vi "art联动采集V4.6.vi"() -> ()   [LabVIEW 2016]
uses:
  <vilib>/Instr/_visa.llb/VISA Configure Serial Port (Instr).vi
  <vilib>/Utility/file.llb/Write Delimited Spreadsheet (DBL).vi
panel:
  in  "分层图查看":bool
  in  "hDevice 2":i32
  in  "逐行扫描":bool
  in  "定位模式":bool
  in  "X终点":dbl
  in  "Y终点":dbl
  in  "高级设置":bool
  in  "Y轴回零速度":dbl=15000.0
  in  "X轴回零速度":dbl=15000.0
  in  "细分设置":dbl=8.0
  in  "等待时间":u32=40
  in  "文件保存":path=path "C:/Users/H301/Desktop/art采集实验数据" caption="保存路径"
  out "行用时（s）":dbl
  out "time（行）":u32
  out "error out":errorcluster caption="错误输出"
  in  "退出扫描(Esc)":bool
  in  "N_Length":i32=16384
  out "M_Length":i32
  out "hDevice":i32=241832032
  out "pulDDR2Length":u32=256
  out "总用时（s）":dbl
  out "毫秒计时值":u32=3586537
  out "数组":dbl[][](array[numeric])=[[58819.77200735986, 88200.32943600747]]
  out "强度图":dbl[][](graph)=[[58819.77200735986, 88200.32943600747]]
  out "judge":dbl
  out "Xloop":dbl
  out "幅频谱":dbl[](graph)
  out "时域谱":dbl[](graph)
  out "错误输出":errorcluster
  in  "启动":bool
  in  "逐点扫描":bool
  in  "X归零":bool
  in  "Y归零":bool
  in  "Y起点":dbl
  in  "Y轴速度":dbl=9000.0
  in  "X轴速度":dbl=9000.0
  out "电机状态":bool
  in  "电机端口":refnum<visa-resource-name>="COM6"
  out "Yloop":dbl=1.0
  out "X扫描范围":dbl=150.0
  out "Y扫描范围":dbl=75.0
  out "Y序":i32
  in  "X起点":dbl
  out "Y(mm)":dbl
  out "x+y 2":dbl=3.0
  in  "Y:":dbl=1.0
  in  "精度":dbl=0.001
  in  "电机急停":bool
  out "X（mm）":dbl
  out "x+y":dbl=1.0
  in  "X:":dbl=1.0
  # "实时坐标"
  # "时域谱"
  # "频域谱"
  # "归零"
  # "扫描区域"
  # "扫描步进(mm)"
  # "X:"
  # "~"
  # "Y:"
  # "~"
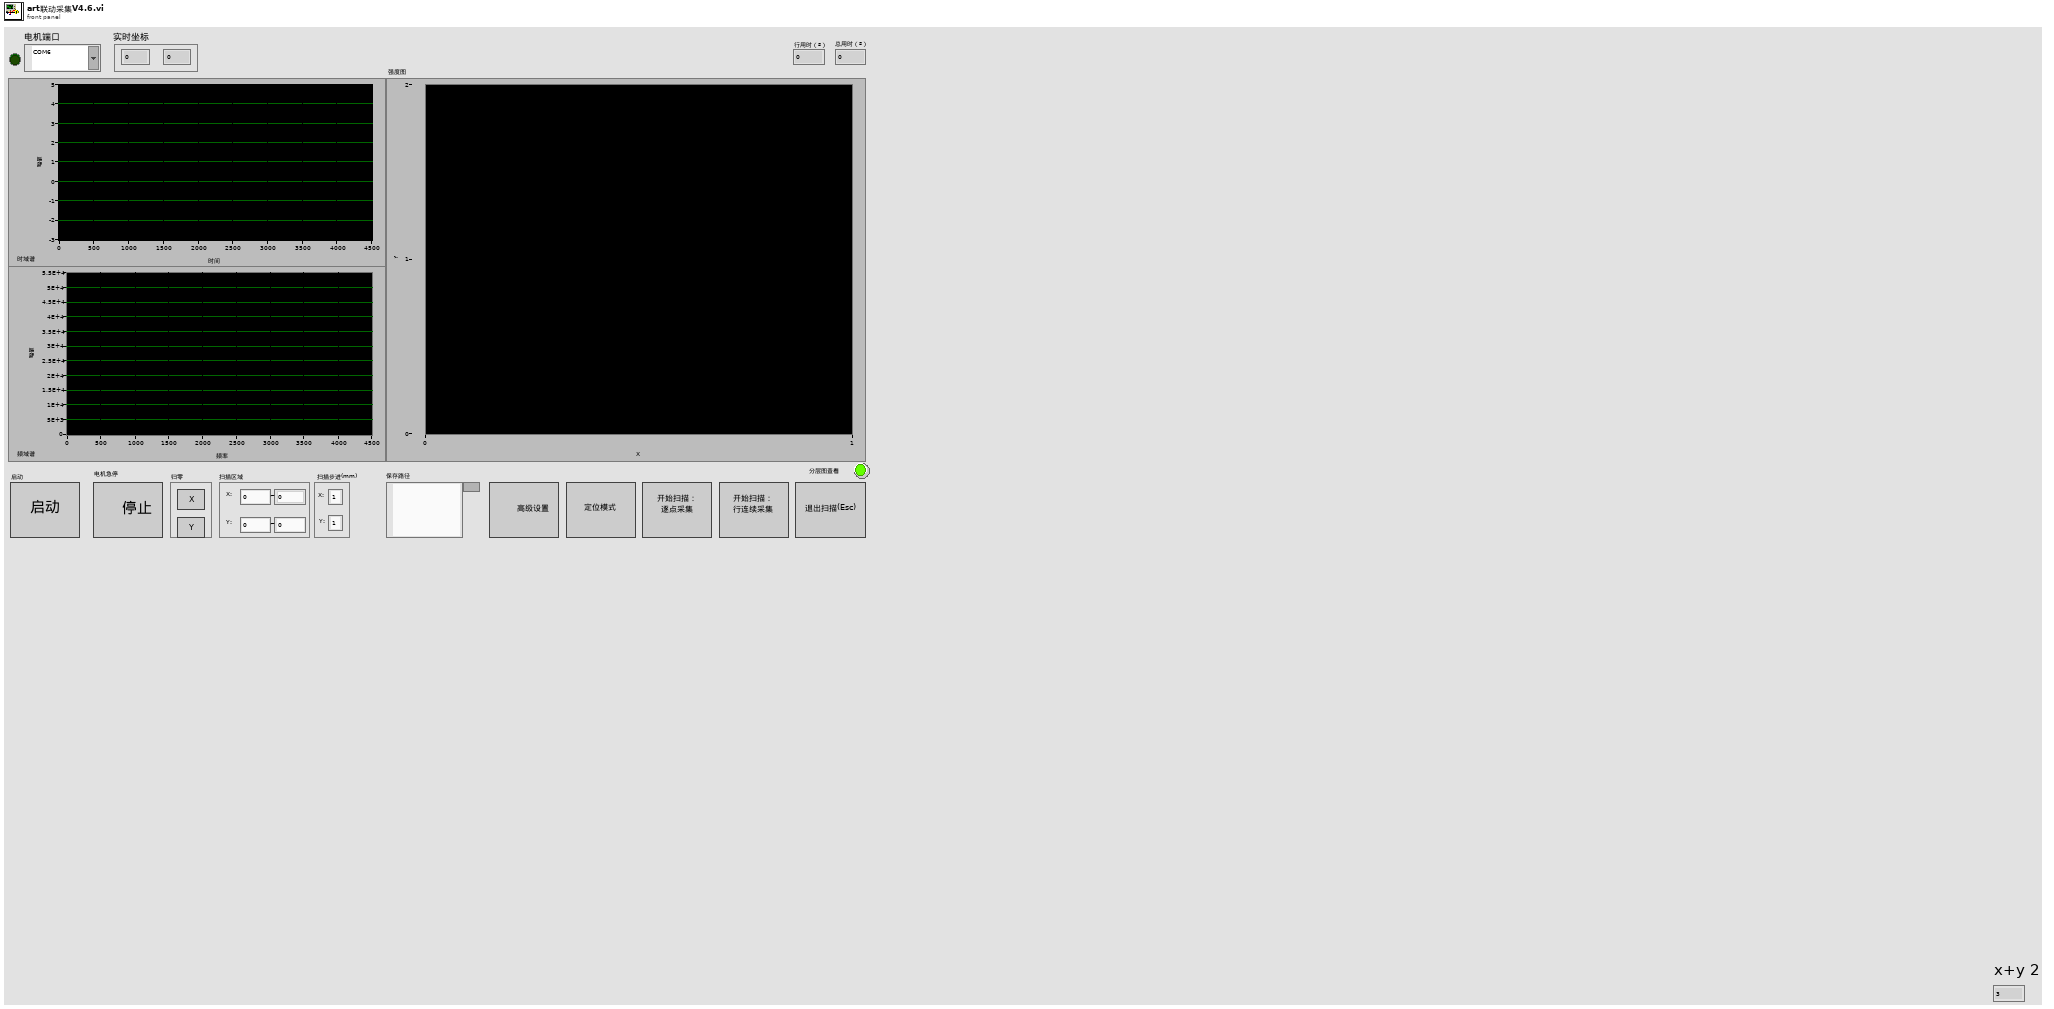
[diagram p1: front panel]
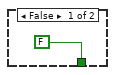
[diagram p2: hidden frame]
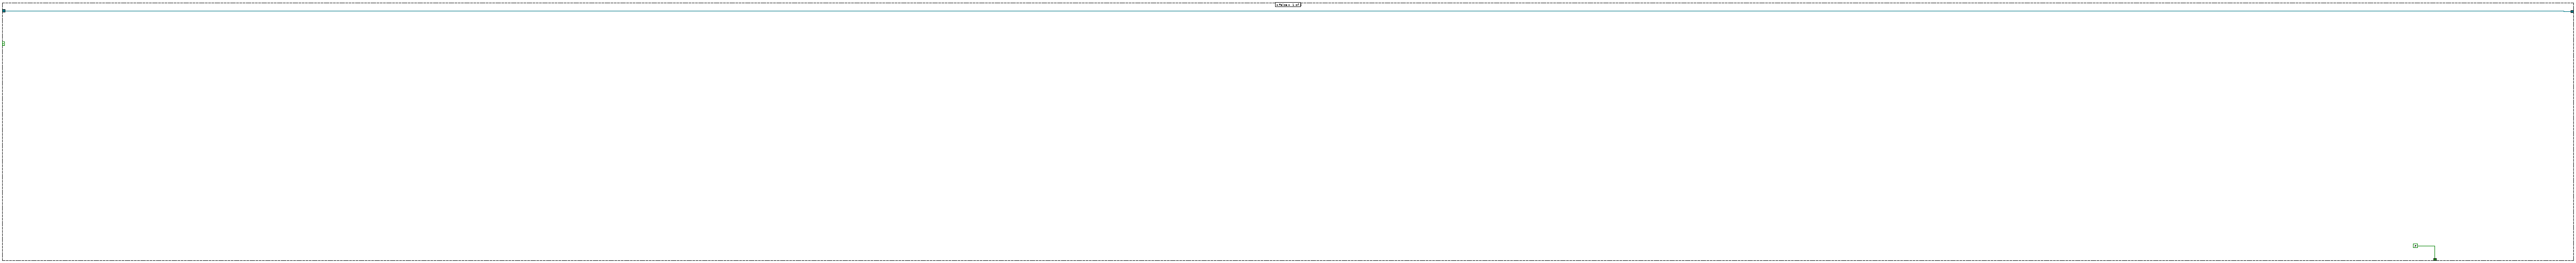
[diagram p3: hidden frame]
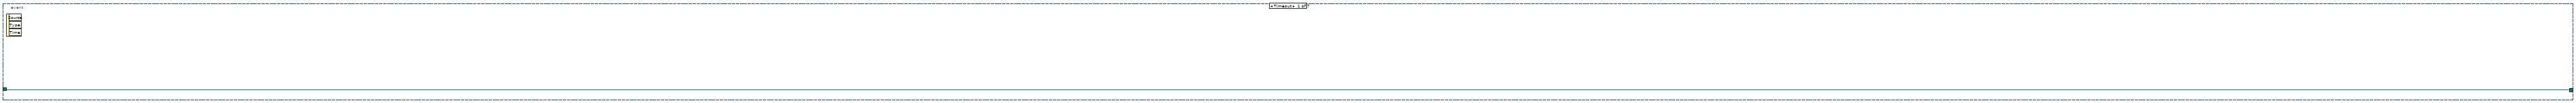
[diagram p4: hidden frame]
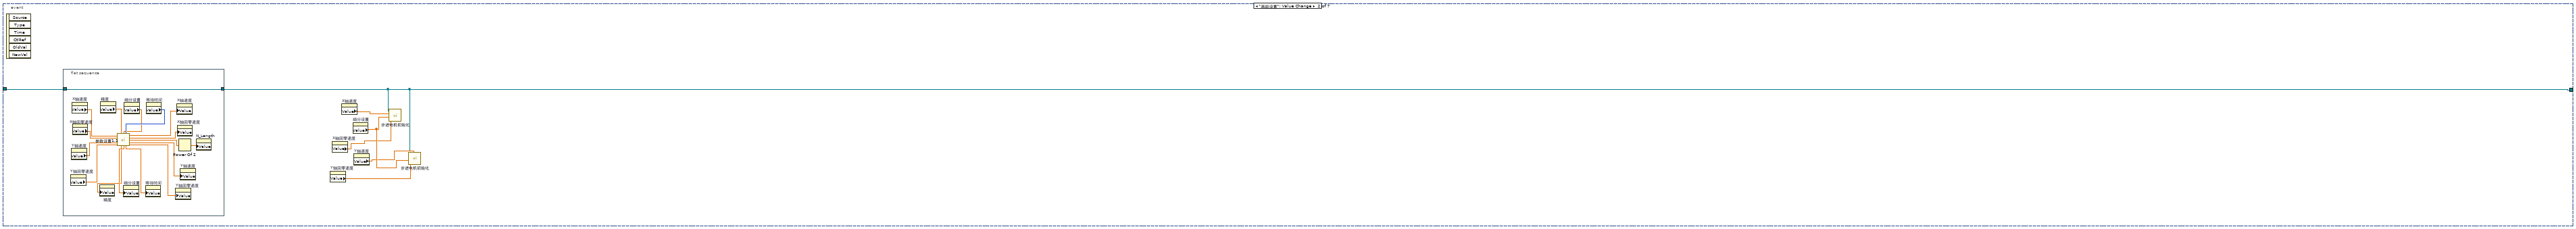
[diagram p5: hidden frame]
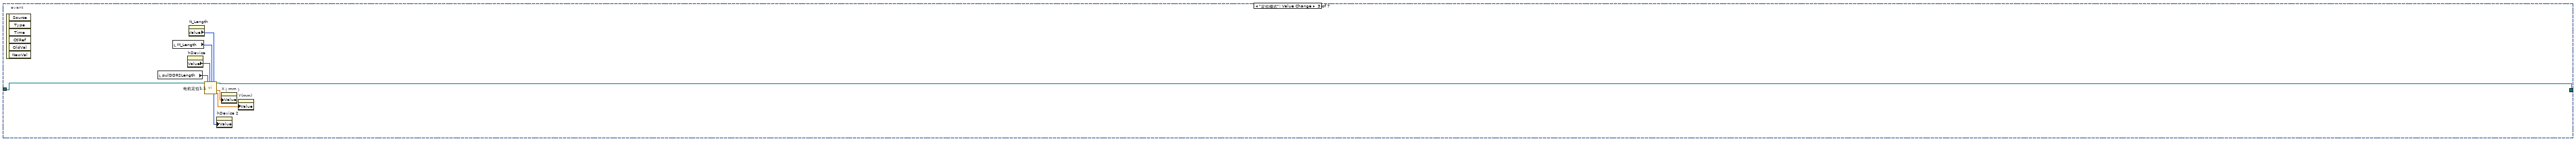
[diagram p6: hidden frame]
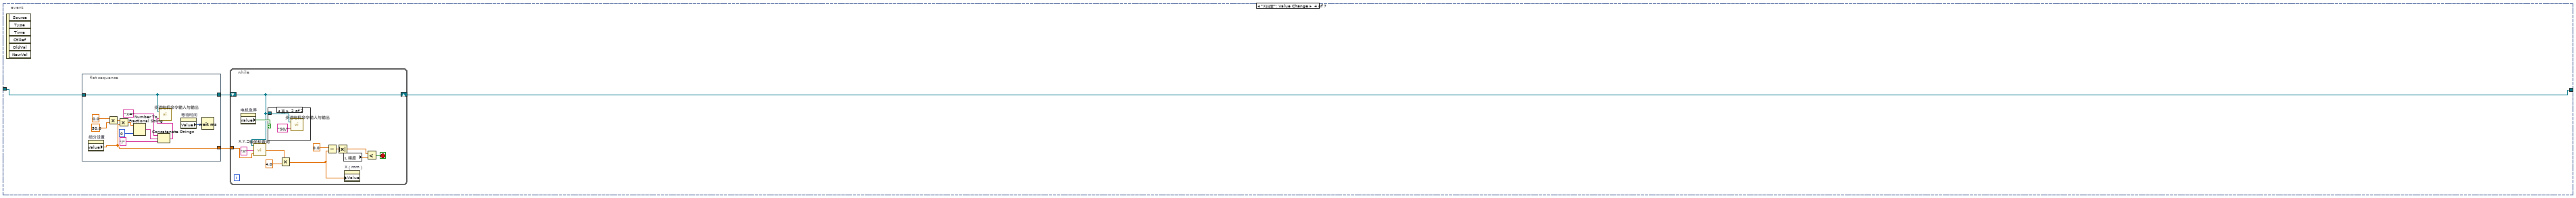
[diagram p7: hidden frame]
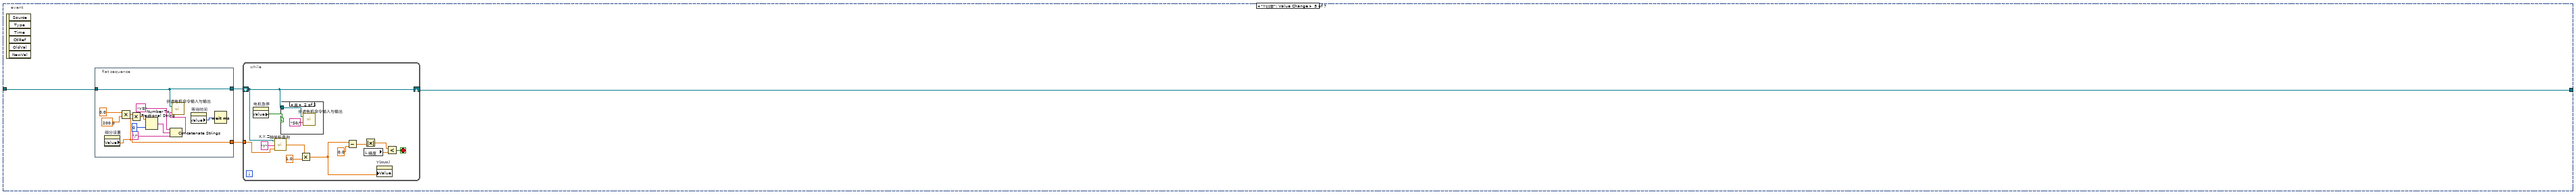
[diagram p9: hidden frame]
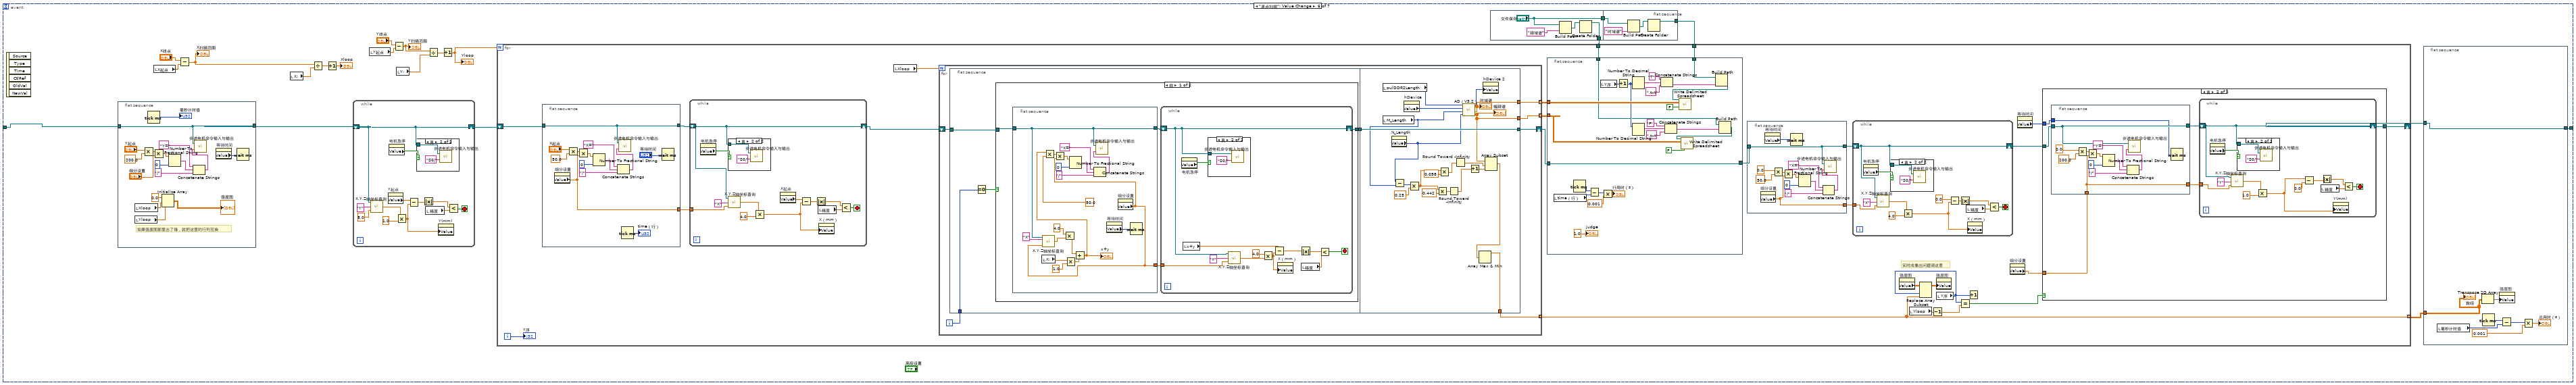
[diagram p11: hidden frame]
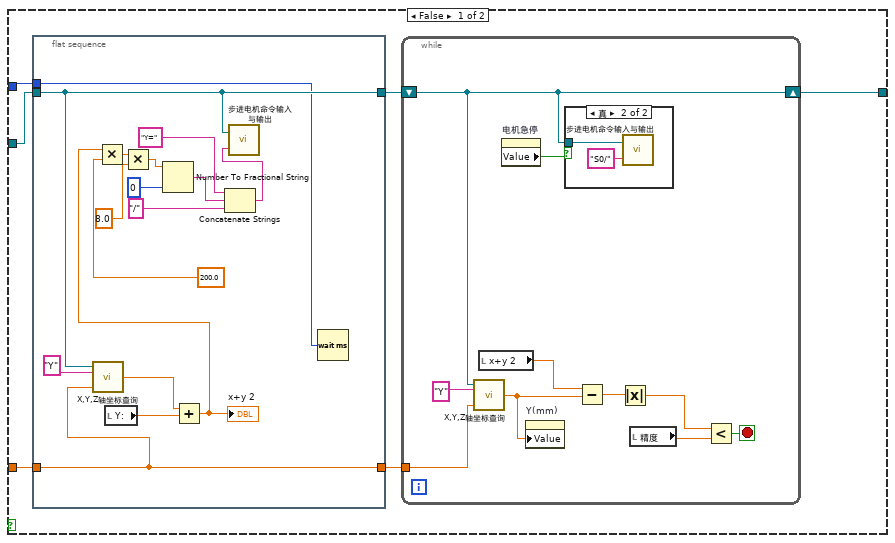
[diagram p15: hidden frame]
diagram:
  n1 = for {
    N: 255 -> [_]
    tunnel: [w10] -> w7 mode=indexing
    i -> [w10]
  }
  n2 = To Unsigned Byte Integer(number=w7) -> (unsigned 8bit integer=w4:u8[])
  n3 = Join Numbers(hi=u16 0, lo=w4) -> ((hi.lo)=w6:u32[])
  n4 = Join Numbers(hi=w4, lo=w4) -> ((hi.lo)=w3:u16[])
  n5 = Join Numbers(hi=w6, lo=w3) -> ((hi.lo)=w2:u64[])
  n6 = property on="强度图" class="IntGraph (严格)"("Color Table"=w2) -> ()  [unwired: 2 in, 2 out]
  n7 = while {
    stop <- w11 stop-if-true
    n8 = case shown="真" "启动" {
      tunnel: [FALSE ("ESC") w20] -> w11
      frame False {
      }
      frame True {
        w33 = 0  # OutClockSource
        w34 = 0  # bClockSourceDir
        w36 = 10000000  # Frequency
        w37 = 0  # ClockSource
        w38 = 0  # TrigLevelVolt
        w26 = 1
        w39 = 0  # TriggerDir
        w40 = 0  # TriggerSource
        w41 = 0  # ATRTriggerChannel
        w42 = 0  # TriggerMode
        w27 = 0  # M_Length
        w43 = 1  # CouplingType
        w44 = 0  # DeviceLgcID
        w54 = u16 0 items=["无", "XON/XOFF", "RTS/CTS", "XON/XOFF & RTS/CTS", "DTR/DSR", "XON/XOFF & DTR/DSR"] ("flow control (0:none)")
        w55 = u16 10 items=["1.0"=10, "1.5"=15, "2.0"=20] ("stop bits (10: 1 bit)")
        # "3"
        # "2"
        # "1"
        n9 = call-poly "VISA Configure Serial Port"("VISA resource name"="电机端口", "baud rate (9600)"=u32 9600, "data bits (8)"=u16 8, "parity (0:none)"=enum16{"None", "Odd", "Even", "Mark", "Space"}."None", "stop bits (10: 1 bit)"=w55, "flow control (0:none)"=w54) -> ("VISA resource name out"=w46:refnum<visa-resource-name>, "error out"=→"error out":errorcluster)  [unwired: 1 in, 7 out]
        n10 = Build Array "InputRange"(w26, w26, w26, w26) -> (w25:i32[])
        n11 = dll-call lib="PTH2aabs CUsersH301Desktopart闭环扫描程序采集卡控制INFamd64PCI8502_32.dll" fn="PCI8502_CreateDevice" label="CreateDevice"("DeviceLgcID"=w44) -> (w31:i32)  [unwired: 4 in, 2 out]
        n12 = property on="细分设置" class="DigNum (严格)"() -> ("Value"=w19:dbl)  [unwired: 2 in, 2 out]
        n13 = Build Array (concatenate) "InitDeviceAD"(w36, w25, w43, w27, "N_Length", w42, w41, w40, w39, w38, w37, w34, w33) -> (w35:i32[])
        n14 = call "步进电机初始化.vi"("回零速度"="X轴回零速度", "细分设置"=w19, "X轴速度"="X轴速度", "串口通信端口"=w46) -> ()  [unwired: 2 in, 1 out]
        n15 = dll-call lib="PTH2aabs CUsersH301Desktopart闭环扫描程序采集卡控制INFamd64PCI8502_32.dll" fn="PCI8502_GetDDR2Length" label="GetDDR2Length"("hDevice"=w31, "pulDDR2Length"=u32 0) -> ("hDevice"=w30:i32, "pulDDR2Length"=→"pulDDR2Length":u32)  [unwired: 4 in, 2 out]
        n16 = call "步进电机初始化.vi"("Y轴速度"="Y轴速度", "回零速度"="Y轴回零速度", "细分设置"=w19, "串口通信端口"=w46) -> ()  [unwired: 2 in, 1 out]
        n17 = call "步进电机命令输入与输出.vi"("输入字符串"="?R/", "串口通信端口"=w46) -> ("返回字符串"=w51:string)
        n18 = dll-call lib="PTH2aabs CUsersH301Desktopart闭环扫描程序采集卡控制INFamd64PCI8502_32.dll" fn="PCI8502_InitDeviceAD" label="InitDeviceAD"("hDevice"=w30, "pADPara"=w35) -> ("hDevice"=→"hDevice":i32)  [unwired: 5 in, 2 out]
        n19 = String Subset(string=w51, offset (0)=0 ("偏移量(0)"), length (rest)=2 ("长度（剩余）")) -> (substring=w48:string)
        n20 = Equal?(x=w48, y="OK") -> (x = y?=w45:bool)
        "电机状态" <- w45
        n21 = case shown="真" w45 {
          tunnel: w46 -> [w61 w64]
          tunnel: [w61 w62] -> w21
          tunnel: [FALSE ("ESC") w63] -> w20
          frame False {
          }
          frame True {
            n22 = while {
              tunnel: ["退出扫描(Esc)"] -> w63
              shift-right: [w65] -> w62
              shift-left: w64 -> [w70]
              stop <- "退出扫描(Esc)" stop-if-true
              n23 = property on="高级设置" class="Bool"("Visible"=TRUE ("可见")) -> ()  [unwired: 2 in, 2 out]
              n24 = property on="定位模式" class="Bool"("Visible"=TRUE ("可见")) -> ()  [unwired: 2 in, 2 out]
              n25 = event shown="[6] \"分层图查看\": 值改变" {
                selector: _ -> [_ _ _ _ _ _ _]
                dyn-events: _ -> [_ _ _ _ _ _ _]
                timeout: 1 -> [_ _ _ _ _ _ _]
                tunnel: w70 -> [w71 w78 w104 w108 w138 w185 w472]
                tunnel: [w71 w72 w103 w106 w136 w179 w471] -> w65
                event Timeout {
                  n26 = event-data() -> ()  [unwired: 1 in, 3 out]
                }
                event "高级设置": Value Change {
                  n27 = event-data() -> ()  [unwired: 1 in, 6 out]
                  n28 = flat-sequence {
                    tunnel: w78 -> [w81]
                    tunnel: [w81] -> w72
                    frame #0 {
                      n29 = property on="Y轴回零速度" class="DigNum (严格)"() -> ("Value"=w85:dbl)  [unwired: 2 in, 2 out]
                      n30 = property on="Y轴速度" class="DigNum (严格)"() -> ("Value"=w84:dbl)  [unwired: 2 in, 2 out]
                      n31 = property on="X轴速度" class="DigNum (严格)"() -> ("Value"=w82:dbl)  [unwired: 2 in, 2 out]
                      n32 = property on="X轴回零速度" class="DigNum (严格)"() -> ("Value"=w83:dbl)  [unwired: 2 in, 2 out]
                      n33 = property on="精度" class="DigNum (严格)"() -> ("Value"=w89:dbl)  [unwired: 2 in, 2 out]
                      n34 = property on="细分设置" class="DigNum (严格)"() -> ("Value"=w90:dbl)  [unwired: 2 in, 2 out]
                      n35 = property on="等待时间" class="DigNum (严格)"() -> ("Value"=w91:u32)  [unwired: 2 in, 2 out]
                      n36 = call "参数设置1.1.vi"("X轴速度"=w82, "精度"=w89, "细分设置"=w90, "等待时间"=w91, "X轴回零速度"=w83, "Y轴速度"=w84, "Y轴回零速度"=w85) -> ("X轴速度"=w92:dbl, "X轴回零速度"=w93:dbl, "采样阶"=w79:dbl, "Y轴速度"=w94:dbl, "精度"=w86:dbl, "细分设置"=w87:dbl, "等待时间"=w88:dbl, "Y轴回零速度"=w95:dbl)  [unwired: 1 in]
                      n37 = property on="精度" class="DigNum (严格)"("Value"=w86) -> ()  [unwired: 2 in, 2 out]
                      n38 = property on="细分设置" class="DigNum (严格)"("Value"=w87) -> ()  [unwired: 2 in, 2 out]
                      n39 = property on="等待时间" class="DigNum (严格)"("Value"=w88) -> ()  [unwired: 2 in, 2 out]
                      n40 = property on="Y轴回零速度" class="DigNum (严格)"("Value"=w95) -> ()  [unwired: 2 in, 2 out]
                      n41 = property on="X轴速度" class="DigNum (严格)"("Value"=w92) -> ()  [unwired: 2 in, 2 out]
                      n42 = property on="X轴回零速度" class="DigNum (严格)"("Value"=w93) -> ()  [unwired: 2 in, 2 out]
                      n43 = Power Of 2(x=w79) -> (2^x=w80:dbl)
                      n44 = property on="Y轴速度" class="DigNum (严格)"("Value"=w94) -> ()  [unwired: 2 in, 2 out]
                      n45 = property on="N_Length" class="DigNum (严格)"("Value"=w80) -> ()  [unwired: 2 in, 2 out]
                    }
                  }
                  n46 = property on="Y轴回零速度" class="DigNum (严格)"() -> ("Value"=w74:dbl)  [unwired: 2 in, 2 out]
                  n47 = property on="X轴回零速度" class="DigNum (严格)"() -> ("Value"=w75:dbl)  [unwired: 2 in, 2 out]
                  n48 = property on="X轴速度" class="DigNum (严格)"() -> ("Value"=w76:dbl)  [unwired: 2 in, 2 out]
                  n49 = property on="细分设置" class="DigNum (严格)"() -> ("Value"=w77:dbl)  [unwired: 2 in, 2 out]
                  n50 = property on="Y轴速度" class="DigNum (严格)"() -> ("Value"=w73:dbl)  [unwired: 2 in, 2 out]
                  n51 = call "步进电机初始化.vi"("回零速度"=w75, "细分设置"=w77, "X轴速度"=w76, "串口通信端口"=w72) -> ()  [unwired: 2 in, 1 out]
                  n52 = call "步进电机初始化.vi"("Y轴速度"=w73, "回零速度"=w74, "细分设置"=w77, "串口通信端口"=w72) -> ()  [unwired: 2 in, 1 out]
                }
                event "定位模式": Value Change {
                  n53 = event-data() -> ()  [unwired: 1 in, 6 out]
                  n54 = local read "pulDDR2Length"() -> (w100:u32)
                  n55 = local read "M_Length"() -> (w98:i32)
                  n56 = property on="hDevice" class="DigNum (严格)"() -> ("Value"=w99:i32)  [unwired: 2 in, 2 out]
                  n57 = property on="N_Length" class="DigNum (严格)"() -> ("Value"=w97:i32)  [unwired: 2 in, 2 out]
                  n58 = call "电机定位1.1.vi"("VISA I"=w104, "pulDDR2Length"=w100, "hDevice"=w99, "M-length"=w98, "N-length"=w97) -> ("hDevice out"=w96:i32, "VISA O"=w103:refnum<visa-resource-name>, "X"=w102:dbl, "Y"=w101:dbl)  [unwired: 11 in]
                  n59 = property on="hDevice 2" class="DigNum (严格)"("Value"=w96) -> ()  [unwired: 2 in, 2 out]
                  n60 = property on="X（mm）" class="DigNum (严格)"("Value"=w102) -> ()  [unwired: 2 in, 2 out]
                  n61 = property on="Y(mm)" class="DigNum (严格)"("Value"=w101) -> ()  [unwired: 2 in, 2 out]
                }
                event "X归零": Value Change {
                  n62 = event-data() -> ()  [unwired: 1 in, 6 out]
                  n63 = flat-sequence {
                    tunnel: w108 -> [w112]
                    tunnel: [w112] -> w107
                    tunnel: [w109] -> w105
                    frame #0 {
                      n64 = property on="细分设置" class="DigNum (严格)"() -> ("Value"=w109:dbl)  [unwired: 2 in, 2 out]
                      n65 = Multiply(x=0.0, y=50.0) -> (x*y=w115:dbl)
                      n66 = Multiply(x=w115, y=w109) -> (x*y=w120:dbl)
                      n67 = Number To Fractional String(number=w120, precision (6)=i16 0 ("精度(6)")) -> (F-format string=w118:string)  [unwired: 2 out]
                      n68 = Concatenate Strings("X=" ("字符串"), w118, "/" ("字符串")) -> (w113:string)
                      n69 = call "步进电机命令输入与输出.vi"("输入字符串"=w113, "串口通信端口"=w112) -> ()  [unwired: 1 out]
                      n70 = property on="等待时间" class="DigNum (严格)"() -> ("Value"=w110:u32)  [unwired: 2 in, 2 out]
                      n71 = Wait (ms)(milliseconds to wait=w110) -> ()  [unwired: 1 out]
                    }
                  }
                  n72 = while {
                    tunnel: w105 -> [w121]
                    shift-right: [w122] -> w106
                    shift-left: w107 -> [w122]
                    stop <- w128 stop-if-true
                    n73 = property on="电机急停" class="Bool (严格)"() -> ("Value"=w129:bool)  [unwired: 2 in, 2 out]
                    n74 = call "X,Y,Z轴坐标查询.vi"("细分设置"=w121, "查询坐标轴"="X", "串口通信端口"=w122) -> ("坐标(mm)"=w130:dbl)
                    n75 = case shown="真" w129 {
                      tunnel: w122 -> [_ w133]
                      frame False {
                      }
                      frame True {
                        n76 = call "步进电机命令输入与输出.vi"("输入字符串"="S0/", "串口通信端口"=w133) -> ()  [unwired: 1 out]
                      }
                    }
                    n77 = Multiply(x=w130, y=4.0 ("x")) -> (x*y=w126:dbl)
                    n78 = Subtract(x=0.0, y=w126) -> (x-y=w125:dbl)
                    n79 = Absolute Value(x=w125) -> (abs(x)=w124:dbl)
                    n80 = local read "精度"() -> (w127:dbl)
                    n81 = property on="X（mm）" class="DigNum (严格)"("Value"=w126) -> ()  [unwired: 2 in, 2 out]
                    n82 = Less?(x=w124, y=w127) -> (x < y?=w128:bool)
                  }
                }
                event "Y归零": Value Change {
                  n83 = event-data() -> ()  [unwired: 1 in, 6 out]
                  n84 = flat-sequence {
                    tunnel: w138 -> [w142]
                    tunnel: [w142] -> w137
                    tunnel: [w139] -> w135
                    frame #0 {
                      n85 = property on="细分设置" class="DigNum (严格)"() -> ("Value"=w139:dbl)  [unwired: 2 in, 2 out]
                      n86 = Multiply(x=0.0, y=200.0) -> (x*y=w145:dbl)
                      n87 = Multiply(x=w145, y=w139) -> (x*y=w150:dbl)
                      n88 = Number To Fractional String(number=w150, precision (6)=i16 0 ("精度(6)")) -> (F-format string=w148:string)  [unwired: 2 out]
                      n89 = Concatenate Strings("Y=" ("字符串"), w148, "/" ("字符串")) -> (w143:string)
                      n90 = call "步进电机命令输入与输出.vi"("输入字符串"=w143, "串口通信端口"=w142) -> ()  [unwired: 1 out]
                      n91 = property on="等待时间" class="DigNum (严格)"() -> ("Value"=w140:u32)  [unwired: 2 in, 2 out]
                      n92 = Wait (ms)(milliseconds to wait=w140) -> ()  [unwired: 1 out]
                    }
                  }
                  n93 = while {
                    tunnel: w135 -> [w151]
                    shift-right: [w152] -> w136
                    shift-left: w137 -> [w152]
                    stop <- w158 stop-if-true
                    n94 = property on="电机急停" class="Bool (严格)"() -> ("Value"=w159:bool)  [unwired: 2 in, 2 out]
                    n95 = call "X,Y,Z轴坐标查询.vi"("细分设置"=w151, "查询坐标轴"="Y", "串口通信端口"=w152) -> ("坐标(mm)"=w160:dbl)
                    n96 = case shown="真" w159 {
                      tunnel: w152 -> [_ w163]
                      frame False {
                      }
                      frame True {
                        n97 = call "步进电机命令输入与输出.vi"("输入字符串"="S0/", "串口通信端口"=w163) -> ()  [unwired: 1 out]
                      }
                    }
                    n98 = Multiply(x=w160, y=1.0 ("x")) -> (x*y=w156:dbl)
                    n99 = Subtract(x=w156, y=0.0 ("x")) -> (x-y=w154:dbl)
                    n100 = local read "精度"() -> (w157:dbl)
                    n101 = Absolute Value(x=w154) -> (abs(x)=w153:dbl)
                    n102 = property on="Y(mm)" class="DigNum (严格)"("Value"=w156) -> ()  [unwired: 2 in, 2 out]
                    n103 = Less?(x=w153, y=w157) -> (x < y?=w158:bool)
                  }
                }
                event "逐点扫描": Value Change {
                  n104 = event-data() -> ()  [unwired: 1 in, 6 out]
                  n105 = flat-sequence {
                    tunnel: w185 -> [w210]
                    tunnel: [w210] -> w175
                    frame #0 {
                      # "如果强度图那里出了错，就把这里的行列互换"
                      n106 = local read "Xloop"() -> (w205:dbl)
                      n107 = local read "Yloop"() -> (w204:dbl)
                      n108 = Multiply(x="Y起点", y=200.0) -> (x*y=w213:dbl)
                      n109 = Tick Count (ms)() -> (millisecond timer value=→"毫秒计时值":u32)
                      n110 = Multiply(x=w213, y="细分设置") -> (x*y=w218:dbl)
                      n111 = Initialize Array(0.0 ("元素"), w205, w204) -> (→"强度图":dbl[][])
                      n112 = Number To Fractional String(number=w218, precision (6)=i16 0 ("精度(6)")) -> (F-format string=w216:string)  [unwired: 2 out]
                      n113 = Concatenate Strings("Y=" ("字符串"), w216, "/" ("字符串")) -> (w211:string)
                      n114 = call "步进电机命令输入与输出.vi"("输入字符串"=w211, "串口通信端口"=w210) -> ()  [unwired: 1 out]
                      n115 = property on="等待时间" class="DigNum (严格)"() -> ("Value"=w202:u32)  [unwired: 2 in, 2 out]
                      n116 = Wait (ms)(milliseconds to wait=w202) -> ()  [unwired: 1 out]
                    }
                  }
                  n117 = local read "X起点"() -> (w171:dbl)
                  n118 = Subtract(x="X终点", y=w171) -> (x-y=w170:dbl)
                  "X扫描范围" <- w170
                  n119 = local read "X:"() -> (w178:dbl)
                  n120 = Divide(x=w170, y=w178) -> (x/y=w176:dbl)
                  n121 = Increment(x=w176) -> (x+1=→"Xloop":dbl)
                  n122 = while {
                    shift-right: [w219] -> w167
                    shift-left: w175 -> [w219]
                    stop <- w224 stop-if-true
                    n123 = call "X,Y,Z轴坐标查询.vi"("细分设置"=8.0, "查询坐标轴"="Y", "串口通信端口"=w219) -> ("坐标(mm)"=w226:dbl)
                    n124 = property on="Y起点" class="DigNum (严格)"() -> ("Value"=w228:dbl)  [unwired: 2 in, 2 out]
                    n125 = property on="电机急停" class="Bool (严格)"() -> ("Value"=w225:bool)  [unwired: 2 in, 2 out]
                    n126 = Multiply(x=w226, y=1.0 ("x")) -> (x*y=w222:dbl)
                    n127 = Subtract(x=w228, y=w222) -> (x-y=w221:dbl)
                    n128 = case shown="真" w225 {
                      tunnel: w219 -> [_ w231]
                      frame False {
                      }
                      frame True {
                        n129 = call "步进电机命令输入与输出.vi"("输入字符串"="S0/", "串口通信端口"=w231) -> ()  [unwired: 1 out]
                      }
                    }
                    n130 = Absolute Value(x=w221) -> (abs(x)=w220:dbl)
                    n131 = local read "精度"() -> (w223:dbl)
                    n132 = property on="Y(mm)" class="DigNum (严格)"("Value"=w222) -> ()  [unwired: 2 in, 2 out]
                    n133 = Less?(x=w220, y=w223) -> (x < y?=w224:bool)
                  }
                  n134 = local read "Y起点"() -> (w173:dbl)
                  n135 = Subtract(x="Y终点", y=w173) -> (x-y=w169:dbl)
                  "Y扫描范围" <- w169
                  n136 = local read "Y:"() -> (w184:dbl)
                  n137 = Divide(x=w169, y=w184) -> (x/y=w183:dbl)
                  n138 = Increment(x=w183) -> (x+1=w182:dbl)
                  "Yloop" <- w182
                  n139 = for {
                    N: w182 -> [_]
                    shift-right: [w255] -> w181
                    shift-left: w167 -> [w235]
                    tunnel: [w237] -> w180 mode=indexing
                    tunnel: w165 -> [w241]
                    tunnel: w168 -> [w240]
                    i -> [w256]
                    # "实时成像出问题调这里"
                    n140 = flat-sequence {
                      tunnel: w235 -> [w313]
                      tunnel: [w313] -> w254
                      tunnel: [w309] -> w245
                      frame #0 {
                        n141 = property on="细分设置" class="DigNum (严格)"() -> ("Value"=w309:dbl)  [unwired: 2 in, 2 out]
                        n142 = Multiply(x="X起点", y=50.0) -> (x*y=w316:dbl)
                        n143 = Multiply(x=w316, y=w309) -> (x*y=w321:dbl)
                        n144 = Number To Fractional String(number=w321, precision (6)=i16 0 ("精度(6)")) -> (F-format string=w319:string)  [unwired: 2 out]
                        n145 = Concatenate Strings("X=" ("字符串"), w319, "/" ("字符串")) -> (w314:string)
                        n146 = call "步进电机命令输入与输出.vi"("输入字符串"=w314, "串口通信端口"=w313) -> ()  [unwired: 1 out]
                        n147 = Tick Count (ms)() -> (millisecond timer value=→"time（行）":u32)
                        n148 = Wait (ms)(milliseconds to wait="等待时间") -> ()  [unwired: 1 out]
                      }
                    }
                    n149 = while {
                      tunnel: w245 -> [w323]
                      shift-right: [w322] -> w233
                      shift-left: w254 -> [w322]
                      stop <- w328 stop-if-true
                      n150 = property on="电机急停" class="Bool (严格)"() -> ("Value"=w329:bool)  [unwired: 2 in, 2 out]
                      n151 = case shown="真" w329 {
                        tunnel: w322 -> [_ w334]
                        frame False {
                        }
                        frame True {
                          n152 = call "步进电机命令输入与输出.vi"("输入字符串"="S0/", "串口通信端口"=w334) -> ()  [unwired: 1 out]
                        }
                      }
                      n153 = call "X,Y,Z轴坐标查询.vi"("细分设置"=w323, "查询坐标轴"="X", "串口通信端口"=w322) -> ("坐标(mm)"=w330:dbl)
                      n154 = Multiply(x=w330, y=4.0 ("x")) -> (x*y=w326:dbl)
                      n155 = property on="X起点" class="DigNum (严格)"() -> ("Value"=w332:dbl)  [unwired: 2 in, 2 out]
                      n156 = Subtract(x=w332, y=w326) -> (x-y=w325:dbl)
                      n157 = Absolute Value(x=w325) -> (abs(x)=w324:dbl)
                      n158 = local read "精度"() -> (w327:dbl)
                      n159 = property on="X（mm）" class="DigNum (严格)"("Value"=w326) -> ()  [unwired: 2 in, 2 out]
                      n160 = Less?(x=w324, y=w327) -> (x < y?=w328:bool)
                    }
                    n161 = local read "Xloop"() -> (w246:dbl)
                    n162 = for {
                      N: w246 -> [_]
                      shift-right: [w407] -> w234
                      shift-left: w233 -> [w402]
                      tunnel: [w406] -> w253 mode=indexing
                      tunnel: [w405] -> w252 mode=indexing
                      tunnel: [w404] -> w237 mode=indexing
                      i -> [w403]
                      n163 = flat-sequence {
                        tunnel: w402 -> [w412]
                        tunnel: [w411] -> w408
                        tunnel: w403 -> [w409]
                        tunnel: [w470] -> w407
                        tunnel: w408 -> [w470]
                        tunnel: [w469] -> w406
                        tunnel: [w468] -> w405
                        tunnel: [w466] -> w404
                        frame #0 {
                          n164 = Equal To 0?(x=w409) -> (x = 0?=w410:bool)
                          n165 = case shown="假" w410 {
                            tunnel: w412 -> [w415 w450]
                            tunnel: [w414 w450] -> w411
                            frame False {
                              n166 = flat-sequence {
                                tunnel: w415 -> [w425]
                                tunnel: [w425] -> w416
                                tunnel: [w417] -> w413
                                frame #0 {
                                n167 = local read "X:"() -> (w419:dbl)
                                n168 = Multiply(x=w419, y=1.0 ("x")) -> (x*y=w424:dbl)
                                n169 = property on="等待时间" class="DigNum (严格)"() -> ("Value"=w418:u32)  [unwired: 2 in, 2 out]
                                n170 = property on="细分设置" class="DigNum (严格)"() -> ("Value"=w417:dbl)  [unwired: 2 in, 2 out]
                                n171 = call "X,Y,Z轴坐标查询.vi"("细分设置"=w417, "查询坐标轴"="X", "串口通信端口"=w425) -> ("坐标(mm)"=w421:dbl)
                                n172 = Multiply(x=4.0, y=w421) -> (x*y=w420:dbl)
                                n173 = Add(x=w420, y=w424) -> (x+y=w427:dbl)
                                "x+y" <- w427
                                n174 = Multiply(x=w427, y=50.0) -> (x*y=w430:dbl)
                                n175 = Multiply(x=w430, y=w417) -> (x*y=w435:dbl)
                                n176 = Number To Fractional String(number=w435, precision (6)=i16 0 ("精度(6)")) -> (F-format string=w433:string)  [unwired: 2 out]
                                n177 = Concatenate Strings("X=" ("字符串"), w433, "/" ("字符串")) -> (w428:string)
                                n178 = call "步进电机命令输入与输出.vi"("输入字符串"=w428, "串口通信端口"=w425) -> ()  [unwired: 1 out]
                                n179 = Wait (ms)(milliseconds to wait=w418) -> ()  [unwired: 1 out]
                                }
                              }
                              n180 = while {
                                tunnel: w413 -> [w436]
                                shift-right: [w445] -> w414
                                shift-left: w416 -> [w445]
                                stop <- w444 stop-if-true
                                n181 = property on="电机急停" class="Bool (严格)"() -> ("Value"=w442:bool)  [unwired: 2 in, 2 out]
                                n182 = local read "x+y"() -> (w446:dbl)
                                n183 = case shown="真" w442 {
                                tunnel: w445 -> [_ w448]
                                frame False {
                                }
                                frame True {
                                n184 = call "步进电机命令输入与输出.vi"("输入字符串"="S0/", "串口通信端口"=w448) -> ()  [unwired: 1 out]
                                }
                                }
                                n185 = call "X,Y,Z轴坐标查询.vi"("细分设置"=w436, "查询坐标轴"="X", "串口通信端口"=w445) -> ("坐标(mm)"=w440:dbl)
                                n186 = Multiply(x=4.0, y=w440) -> (x*y=w439:dbl)
                                n187 = Subtract(x=w446, y=w439) -> (x-y=w438:dbl)
                                n188 = property on="X（mm）" class="DigNum (严格)"("Value"=w439) -> ()  [unwired: 2 in, 2 out]
                                n189 = Absolute Value(x=w438) -> (abs(x)=w437:dbl)
                                n190 = local read "精度"() -> (w441:dbl)
                                n191 = Less?(x=w437, y=w441) -> (x < y?=w444:bool)
                              }
                            }
                            frame True {
                            }
                          }
                        }
                        frame #1 {
                          n192 = local read "pulDDR2Length"() -> (w465:u32)
                          n193 = local read "M_Length"() -> (w464:i32)
                          n194 = property on="N_Length" class="DigNum (严格)"() -> ("Value"=w453:i32)  [unwired: 2 in, 2 out]
                          n195 = Subtract(x=w453, y=w464) -> (x-y=w462:i32)
                          n196 = property on="hDevice" class="DigNum (严格)"() -> ("Value"=w451:i32)  [unwired: 2 in, 2 out]
                          n197 = Multiply(x=w462, y=0.25) -> (x*y=w455:dbl)
                          n198 = Multiply(x=w455, y=0.442) -> (x*y=w457:dbl)
                          n199 = Multiply(x=w455, y=0.058) -> (x*y=w459:dbl)
                          n200 = Round Toward -Infinity(1:w457) -> (0:w454:dbl)
                          n201 = Round Toward -Infinity(1:w459) -> (0:w458:dbl)
                          n202 = call "AD（V3.2）.vi"("N-length"=w453, "M-length"=w464, "hDevice"=w451, "pulDDR2Length"=w465) -> ("幅频谱"=w468:dbl[], "时域谱"=w469:dbl[], "hDevice out"=w452:i32)  [unwired: 5 in]
                          "时域谱" <- w469
                          "幅频谱" <- w468
                          n203 = Increment(x=w454) -> (x+1=w461:dbl)
                          n204 = property on="hDevice 2" class="DigNum (严格)"("Value"=w452) -> ()  [unwired: 2 in, 2 out]
                          n205 = Array Subset(array=w468, index=w458, length=w461) -> (w467:dbl[])
                          n206 = Array Max & Min(array=w467) -> (max value=w466:dbl)  [unwired: 3 out]
                        }
                      }
                    }
                    n207 = flat-sequence {
                      tunnel: w252 -> [w290]
                      tunnel: w253 -> [w298]
                      tunnel: w234 -> [w307]
                      tunnel: [w307] -> w248
                      tunnel: w241 -> [w285]
                      tunnel: w240 -> [w284]
                      frame #0 {
                        n208 = local read "time（行）"() -> (w306:u32)
                        n209 = Tick Count (ms)() -> (millisecond timer value=w302:u32)
                        n210 = Subtract(x=w302, y=w306) -> (x-y=w305:u32)
                        n211 = local read "Y序"() -> (w286:i32)
                        n212 = Multiply(x=w305, y=0.001) -> (x*y=→"行用时（s）":dbl)
                        n213 = Increment(x=w286) -> (x+1=w287:i32)
                        n214 = Number To Decimal String(number=w287) -> (decimal integer string=w296:string)  [unwired: 1 in]
                        n215 = Number To Decimal String(number=w287) -> (decimal integer string=w295:string)  [unwired: 1 in]
                        n216 = Concatenate Strings("T" ("字符串"), w296, ".txt" ("字符串")) -> (w299:string)
                        n217 = Concatenate Strings("F" ("字符串"), w295, ".txt" ("字符串")) -> (w293:string)
                        n218 = Build Path(base path=w285, name or relative path=w299) -> (appended path=w301:path)
                        n219 = call-poly <vilib>:"Write Delimited Spreadsheet.vi"("file path (dialog if empty)"=w301, "2D data"=w298, "transpose? (no:F)"=FALSE) -> ()  [unwired: 11 in, 2 out]
                        n220 = Build Path(base path=w284, name or relative path=w293) -> (appended path=w291:path)
                        n221 = call-poly <vilib>:"Write Delimited Spreadsheet.vi"("file path (dialog if empty)"=w291, "2D data"=w290, "transpose? (no:F)"=FALSE) -> ()  [unwired: 11 in, 2 out]
                        "judge" <- 1.0
                      }
                    }
                    n222 = flat-sequence {
                      tunnel: w248 -> [w261]
                      tunnel: [w261] -> w249
                      tunnel: [w259] -> w244
                      frame #0 {
                        n223 = property on="细分设置" class="DigNum (严格)"() -> ("Value"=w259:dbl)  [unwired: 2 in, 2 out]
                        n224 = property on="等待时间" class="DigNum (严格)"() -> ("Value"=w258:u32)  [unwired: 2 in, 2 out]
                        n225 = Multiply(x=0.0, y=50.0) -> (x*y=w264:dbl)
                        n226 = Multiply(x=w264, y=w259) -> (x*y=w269:dbl)
                        n227 = Wait (ms)(milliseconds to wait=w258) -> ()  [unwired: 1 out]
                        n228 = Number To Fractional String(number=w269, precision (6)=i16 0 ("精度(6)")) -> (F-format string=w267:string)  [unwired: 2 out]
                        n229 = Concatenate Strings("X=" ("字符串"), w267, "/" ("字符串")) -> (w262:string)
                        n230 = call "步进电机命令输入与输出.vi"("输入字符串"=w262, "串口通信端口"=w261) -> ()  [unwired: 1 out]
                      }
                    }
                    n231 = while {
                      tunnel: w244 -> [w270]
                      shift-right: [w271] -> w247
                      shift-left: w249 -> [w271]
                      stop <- w277 stop-if-true
                      n232 = property on="电机急停" class="Bool (严格)"() -> ("Value"=w278:bool)  [unwired: 2 in, 2 out]
                      n233 = call "X,Y,Z轴坐标查询.vi"("细分设置"=w270, "查询坐标轴"="X", "串口通信端口"=w271) -> ("坐标(mm)"=w279:dbl)
                      n234 = case shown="真" w278 {
                        tunnel: w271 -> [_ w282]
                        frame False {
                        }
                        frame True {
                          n235 = call "步进电机命令输入与输出.vi"("输入字符串"="S0/", "串口通信端口"=w282) -> ()  [unwired: 1 out]
                        }
                      }
                      n236 = Multiply(x=w279, y=4.0 ("x")) -> (x*y=w275:dbl)
                      n237 = Subtract(x=0.0, y=w275) -> (x-y=w274:dbl)
                      n238 = Absolute Value(x=w274) -> (abs(x)=w273:dbl)
                      n239 = local read "精度"() -> (w276:dbl)
                      n240 = property on="X（mm）" class="DigNum (严格)"("Value"=w275) -> ()  [unwired: 2 in, 2 out]
                      n241 = Less?(x=w273, y=w276) -> (x < y?=w277:bool)
                    }
                    n242 = property on="强度图" class="IntGraph (严格)"() -> ("Value"=w238:dbl[][])  [unwired: 2 in, 2 out]
                    n243 = local read "Yloop"() -> (w250:dbl)
                    n244 = Decrement(x=w250) -> (x-1=w251:dbl)
                    n245 = local read "Y序"() -> (w236:i32)
                    n246 = Replace Array Subset(array=w238, new element=w237, index (col)=w236) -> (w239:dbl[][])  [unwired: 1 in]
                    n247 = property on="强度图" class="IntGraph (严格)"("Value"=w239) -> ()  [unwired: 2 in, 2 out]
                    n248 = Equal?(x=w236, y=w251) -> (x = y?=w257:bool)
                    n249 = Increment(x=w236) -> ()  [unwired: 1 out]
                    n250 = property on="细分设置" class="DigNum (严格)"() -> ("Value"=w242:dbl)  [unwired: 2 in, 2 out]
                    n251 = property on="等待时间" class="DigNum (严格)"() -> ("Value"=w243:u32)  [unwired: 2 in, 2 out]
                    n252 = case shown="真" w257 {
                      tunnel: w247 -> [w341 w373]
                      tunnel: [w339 w374] -> w255
                      tunnel: w243 -> [w337 w371]
                      tunnel: w242 -> [w336 w370]
                      frame False {
                        n253 = flat-sequence {
                          tunnel: w341 -> [w344]
                          tunnel: [w344] -> w340
                          tunnel: [w342] -> w338
                          tunnel: w337 -> [w343]
                          tunnel: w336 -> [w342]
                          frame #0 {
                            n254 = call "X,Y,Z轴坐标查询.vi"("细分设置"=w342, "查询坐标轴"="Y", "串口通信端口"=w344) -> ("坐标(mm)"=w346:dbl)
                            n255 = local read "Y:"() -> (w345:dbl)
                            n256 = Add(x=w346, y=w345) -> (x+y=w348:dbl)
                            "x+y 2" <- w348
                            n257 = Multiply(x=w348, y=200.0) -> (x*y=w352:dbl)
                            n258 = Multiply(x=w352, y=8.0 ("细分设置")) -> (x*y=w357:dbl)
                            n259 = Number To Fractional String(number=w357, precision (6)=i16 0 ("精度(6)")) -> (F-format string=w355:string)  [unwired: 2 out]
                            n260 = Concatenate Strings("Y=" ("字符串"), w355, "/" ("字符串")) -> (w350:string)
                            n261 = call "步进电机命令输入与输出.vi"("输入字符串"=w350, "串口通信端口"=w344) -> ()  [unwired: 1 out]
                            n262 = Wait (ms)(milliseconds to wait=w343) -> ()  [unwired: 1 out]
                          }
                        }
                        n263 = while {
                          tunnel: w338 -> [w358]
                          shift-right: [w359] -> w339
                          shift-left: w340 -> [w359]
                          stop <- w365 stop-if-true
                          n264 = call "X,Y,Z轴坐标查询.vi"("细分设置"=w358, "查询坐标轴"="Y", "串口通信端口"=w359) -> ("坐标(mm)"=w363:dbl)
                          n265 = local read "x+y 2"() -> (w366:dbl)
                          n266 = property on="电机急停" class="Bool (严格)"() -> ("Value"=w362:bool)  [unwired: 2 in, 2 out]
                          n267 = property on="Y(mm)" class="DigNum (严格)"("Value"=w363) -> ()  [unwired: 2 in, 2 out]
                          n268 = case shown="真" w362 {
                            tunnel: w359 -> [_ w368]
                            frame False {
                            }
                            frame True {
                              n269 = call "步进电机命令输入与输出.vi"("输入字符串"="S0/", "串口通信端口"=w368) -> ()  [unwired: 1 out]
                            }
                          }
                          n270 = Subtract(x=w366, y=w363) -> (x-y=w361:dbl)
                          n271 = Absolute Value(x=w361) -> (abs(x)=w360:dbl)
                          n272 = local read "精度"() -> (w364:dbl)
                          n273 = Less?(x=w360, y=w364) -> (x < y?=w365:bool)
                        }
                      }
                      frame True {
                        n274 = flat-sequence {
                          tunnel: [w378] -> _
                          tunnel: [w378] -> w375
                          tunnel: w373 -> [w378]
                          tunnel: [w376] -> w372
                          tunnel: w371 -> [w377]
                          tunnel: w370 -> [w376]
                          frame #0 {
                            n275 = Multiply(x=0.0, y=200.0) -> (x*y=w382:dbl)
                            n276 = Multiply(x=w382, y=w376) -> (x*y=w387:dbl)
                            n277 = Number To Fractional String(number=w387, precision (6)=i16 0 ("精度(6)")) -> (F-format string=w385:string)  [unwired: 2 out]
                            n278 = Concatenate Strings("Y=" ("字符串"), w385, "/" ("字符串")) -> (w380:string)
                            n279 = call "步进电机命令输入与输出.vi"("输入字符串"=w380, "串口通信端口"=w378) -> ()  [unwired: 1 out]
                            n280 = Wait (ms)(milliseconds to wait=w377) -> ()  [unwired: 1 out]
                          }
                        }
                        n281 = while {
                          tunnel: w372 -> [w388]
                          shift-right: [w389] -> w374
                          shift-left: w375 -> [w389]
                          stop <- w395 stop-if-true
                          n282 = property on="电机急停" class="Bool (严格)"() -> ("Value"=w396:bool)  [unwired: 2 in, 2 out]
                          n283 = call "X,Y,Z轴坐标查询.vi"("细分设置"=w388, "查询坐标轴"="Y", "串口通信端口"=w389) -> ("坐标(mm)"=w397:dbl)
                          n284 = case shown="真" w396 {
                            tunnel: w389 -> [_ w400]
                            frame False {
                            }
                            frame True {
                              n285 = call "步进电机命令输入与输出.vi"("输入字符串"="S0/", "串口通信端口"=w400) -> ()  [unwired: 1 out]
                            }
                          }
                          n286 = Multiply(x=w397, y=1.0 ("x")) -> (x*y=w393:dbl)
                          n287 = Subtract(x=w393, y=0.0 ("x")) -> (x-y=w391:dbl)
                          n288 = local read "精度"() -> (w394:dbl)
                          n289 = Absolute Value(x=w391) -> (abs(x)=w390:dbl)
                          n290 = property on="Y(mm)" class="DigNum (严格)"("Value"=w393) -> ()  [unwired: 2 in, 2 out]
                          n291 = Less?(x=w390, y=w394) -> (x < y?=w395:bool)
                        }
                      }
                    }
                    "Y序" <- w256
                  }
                  n292 = flat-sequence {
                    tunnel: [w186] -> w168
                    tunnel: ["文件保存"] -> w166
                    tunnel: w166 -> [w191]
                    tunnel: [w190] -> w165
                    frame #0 {
                      n293 = Build Path(base path="文件保存", name or relative path="频域谱" ("名称或相对路径")) -> (appended path=w189:path)
                      n294 = Create Folder(path (use dialog)=w189) -> (created path=w186:path)  [unwired: 2 in, 2 out]
                    }
                    frame #1 {
                      n295 = Build Path(base path=w191, name or relative path="时域谱" ("名称或相对路径")) -> (appended path=w192:path)
                      n296 = Create Folder(path (use dialog)=w192) -> (created path=w190:path)  [unwired: 2 in, 2 out]
                    }
                  }
                  n297 = flat-sequence {
                    tunnel: w181 -> [w196]
                    tunnel: w180 -> [w195]
                    tunnel: [w196] -> w179
                    frame #0 {
                      n298 = local read "毫秒计时值"() -> (w200:u32)
                      n299 = Transpose 2D Array(2D array=w195) -> (transposed array=w194:dbl[][])
                      n300 = Tick Count (ms)() -> (millisecond timer value=w201:u32)
                      n301 = property on="强度图" class="IntGraph (严格)"("Value"=w194) -> ()  [unwired: 2 in, 2 out]
                      n302 = Subtract(x=w201, y=w200) -> (x-y=w197:u32)
                      n303 = Multiply(x=w197, y=0.001) -> (x*y=→"总用时（s）":dbl)
                      "数组" <- w195
                    }
                  }
                }
                event "分层图查看": Value Change {
                  n304 = event-data() -> ()  [unwired: 1 in, 6 out]
                  n305 = call "分层图显示1.1.vi"("IN"=w472) -> ("OUT"=w471:string)  [unwired: 10 in]
                }
              }
            }
          }
        }
        n306 = dll-call lib="PTH2]abs CUsersH301Desktopart闭环扫描程序采集卡控制INFamd64\nPCI8502_32" fn="PCI8502_ReleaseDeviceAD" label="ReleaseDeviceAD"("hDevice"="hDevice 2") -> ("hDevice"=w23:i32)  [unwired: 4 in, 2 out]
        n307 = VISA Close(VISA resource name=w21) -> (error out=→"错误输出":errorcluster)  [unwired: 1 in]
        n308 = dll-call lib="PTH2]abs CUsersH301Desktopart闭环扫描程序采集卡控制INFamd64\nPCI8502_32" fn="PCI8502_ReleaseDevice" label="ReleaseDevice"("hDevice"=w23) -> ()  [unwired: 5 in, 2 out]
        "M_Length" <- w27
      }
    }
  }
  n309 = property on="高级设置" class="Bool"("Visible"=FALSE ("可见")) -> ()  [unwired: 2 in, 2 out]
  n310 = property on="定位模式" class="Bool"("Visible"=FALSE ("可见")) -> ()  [unwired: 2 in, 2 out]
